vi "pack2bytes.vi"(1 "Decimal In":u16) -> (0 "Bytes out":u16[](array[numeric]) format="%x")   [LabVIEW 2020]
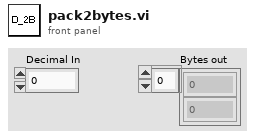
[diagram p1: front panel]
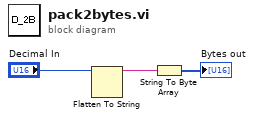
[diagram p0: block diagram]
diagram:
  n1 = Flatten To String(anything="Decimal In") -> (data string=w1:string)  [unwired: 3 in, 2 out]
  n2 = String To Byte Array(string=w1) -> (unsigned byte array=→"Bytes out":u8[])
